vi "test_doubleStopShouldReturnNoError.vi"(11 "Test Case In":refnum<class "TaskControllerTests.lvclass">) -> (0 "error out":errorcluster, 3 "Test Case Out":refnum<class "TaskControllerTests.lvclass">)   [LabVIEW 2023, in "TaskControllerTests.lvclass"]
uses:
  TaskControllerTests.lvclass
  TaskControllerTests.lvclass/TaskControllerTests.ctl
  TaskMock/TaskMock.lvclass
  <vilib>/Astemes/LUnit/Test Case.lvclass
  source/TaskController/TaskController.lvclass
  C:/projects/TLC_Daemon/tests/TaskMock/TaskMock.lvclass
  C:/projects/TLC_Daemon/source/ITask/ITask.lvclass
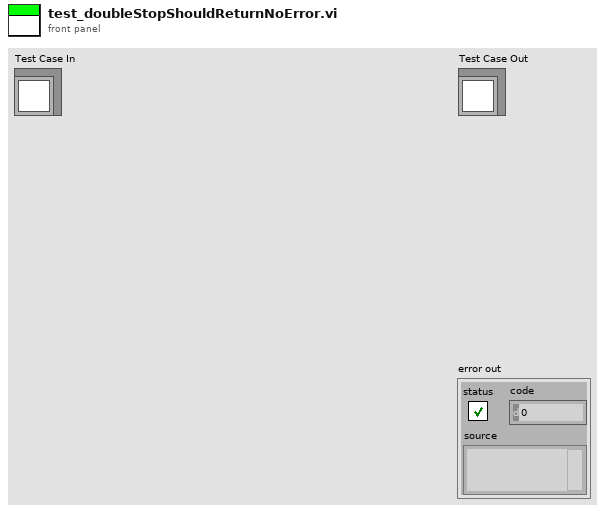
[diagram p1: front panel]
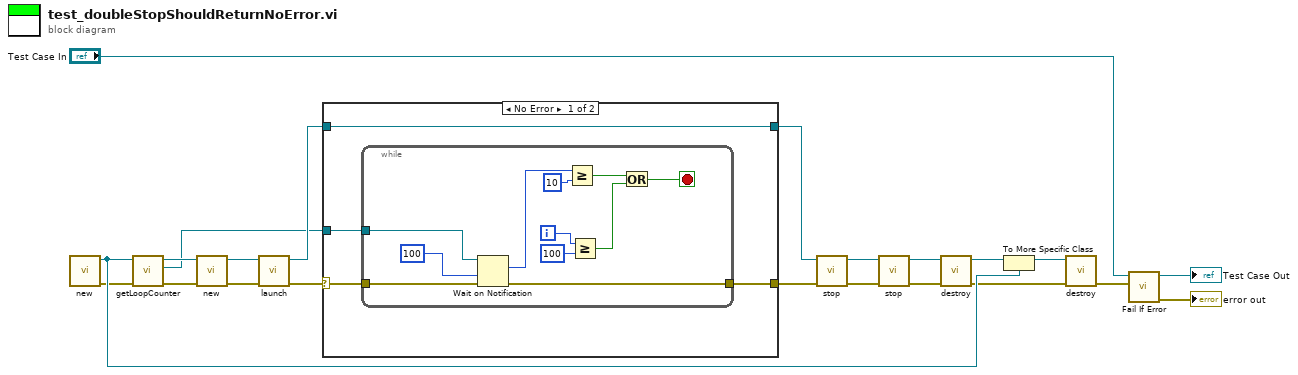
[diagram p0: block diagram]
diagram:
  n1 = call "new.vi"() -> ("error out"=w7:errorcluster, "TaskMock out"=w11:refnum<class "TaskMock.lvclass">)  [unwired: 10 in]
  n2 = call "getLoopCounter.vi"("error in (no error)"=w7, "TaskMock in"=w11) -> ("error out"=w6:errorcluster, "loopCounter"=w14:refnum<notifier>, "TaskMock out"=w15:refnum<class "TaskMock.lvclass">)  [unwired: 7 in]
  n3 = call "new.vi"("error in (no error)"=w6, "task"=w15) -> ("error out"=w18:errorcluster, "TaskController out"=w19:refnum<class "TaskController.lvclass">)  [unwired: 8 in]
  n4 = call "launch.vi"("error in (no error)"=w18, "TaskController in"=w19) -> ("error out"=w16:errorcluster, "TaskController out"=w17:refnum<class "TaskController.lvclass">)  [unwired: 8 in]
  n5 = case shown="No Error" w16 {
    selector: w16 -> [w26 _]
    tunnel: w17 -> [w24 w38]
    tunnel: w14 -> [w25 _]
    tunnel: [w24 w38] -> w13
    tunnel: [w23 _] -> w12
    frame No Error {
      n6 = while {
        tunnel: w26 -> [w28]
        tunnel: w25 -> [w37]
        tunnel: [w27] -> w23
        i -> [w33]
        stop <- w30 stop-if-true
        n7 = Wait on Notification(notifier=w37, timeout in ms (-1)=100, error in (no error)=w28) -> (notification=w35:i32, error out=w27:errorcluster)  [unwired: 1 in, 2 out]
        n8 = Greater Or Equal?(x=w35, y=10) -> (x >= y?=w31:bool)
        n9 = Greater Or Equal?(x=w33, y=100) -> (x >= y?=w29:bool)
        n10 = Or(x=w31, y=w29) -> (x .or. y?=w30:bool)
      }
    }
    frame Error {
    }
  }
  n11 = call "stop.vi"("error in (no error)"=w12, "TaskController in"=w13) -> ("error out"=w5:errorcluster, "TaskController out"=w3:refnum<class "TaskController.lvclass">)  [unwired: 8 in]
  n12 = call "stop.vi"("error in (no error)"=w5, "TaskController in"=w3) -> ("error out"=w4:errorcluster, "TaskController out"=w2:refnum<class "TaskController.lvclass">)  [unwired: 8 in]
  n13 = call "destroy.vi"("error in (no error)"=w4, "TaskController in"=w2) -> ("error out"=w10:errorcluster, "task"=w9:refnum<class "ITask.lvclass">)  [unwired: 8 in]
  n14 = To More Specific Class(target class=w11, reference=w9) -> (specific class reference=w8:refnum<class "TaskMock.lvclass">)  [unwired: 1 in, 1 out]
  n15 = call "destroy.vi"("error in (no error)"=w10, "TaskMock in"=w8) -> ("error out"=w1:errorcluster)  [unwired: 9 in]
  n16 = call <vilib>:"Fail If Error.vi"("Assert error"=w1, "LUnit Test Case In"="Test Case In") -> ("error out"=→"error out":errorcluster, "LUnit Test Case Out"=→"Test Case Out":refnum<class "TaskControllerTests.lvclass">)  [unwired: 8 in]
